vi "Verify File Path.vi"(7 "Default Path":path, 8 "error in":errorcluster, 11 "File Name or Path":string) -> (0 "error out":errorcluster, 3 "File":path, 5 "Stripped Path":path)   [LabVIEW 2021, in "File_CIF_U.lvlib"]
uses:
  File_CIF_U.lvlib
  typedef/File Errors.ctl
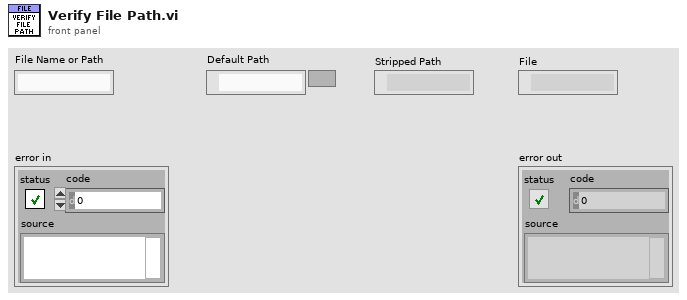
[diagram p1: front panel]
types:
  T1 = typedef "File_CIF_U.lvlib/File Errors.ctl" = enum16{"Invalid File Path"}
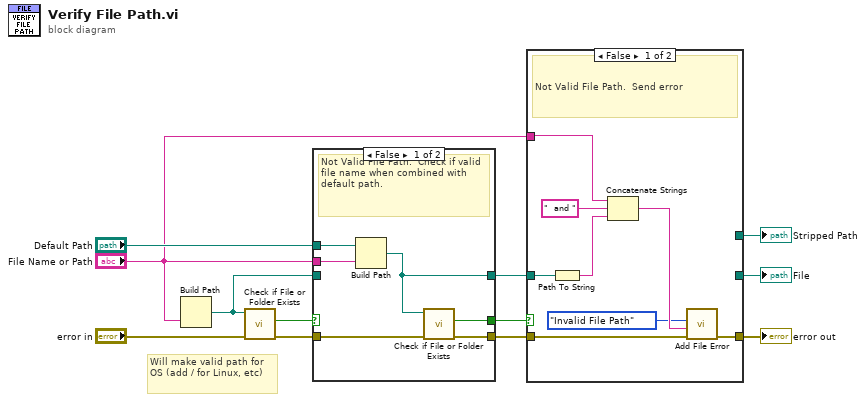
[diagram p0: block diagram]
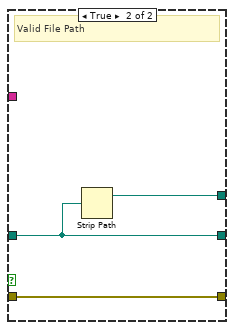
[diagram p2: hidden frame]
diagram:
  # "Will make valid path for OS (add / for Linux, etc)"
  n1 = Build Path(name or relative path="File Name or Path") -> (appended path=w9:path)  [unwired: 1 in]
  n2 = call <vilib>:"Check if File or Folder Exists.vi"("error in (no error)"="error in", "path"=w9) -> ("error out"=w8:errorcluster, "file or folder exists?"=w10:bool)  [unwired: 7 in, 1 out]
  n3 = case shown="False" w10 {
    selector: w10 -> [_ w19]
    tunnel: w9 -> [_ w21]
    tunnel: "File Name or Path" -> [w18 _]
    tunnel: "Default Path" -> [w17 _]
    tunnel: w8 -> [w16 w20]
    tunnel: [w15 w20] -> w7
    tunnel: [w14 w19] -> w6
    tunnel: [w13 w21] -> w5
    frame False {
      # "Not Valid File Path.  Check if valid file name when combined with default path."
      n4 = Build Path(base path=w17, name or relative path=w18) -> (appended path=w13:path)
      n5 = call <vilib>:"Check if File or Folder Exists.vi"("error in (no error)"=w16, "path"=w13) -> ("error out"=w15:errorcluster, "file or folder exists?"=w14:bool)  [unwired: 7 in, 1 out]
    }
    frame True {
      # "Valid File Path"
    }
  }
  n6 = case shown="False" w6 {
    tunnel: w5 -> [w27 w31]
    tunnel: w7 -> [w29 w32]
    tunnel: [w28 w32] -> w1
    tunnel: [_ w31] -> w4
    tunnel: [_ w30] -> w3
    tunnel: "File Name or Path" -> [w26 _]
    frame False {
      # "Not Valid File Path.  Send error"
      n7 = Path To String(path=w27) -> (string=w24:string)
      n8 = Concatenate Strings(w26, "  and " ("string"), w24) -> (w23:string)
      n9 = call "Add File Error.vi"("error in (no error)"=w29, "String to Append"=w23, "Error"=File_Errors."Invalid File Path") -> ("error out"=w28:errorcluster)  [unwired: 8 in]
    }
    frame True {
      # "Valid File Path"
      n10 = Strip Path(path=w31) -> (stripped path=w30:path)  [unwired: 1 out]
    }
  }
  "File" <- w4
  "Stripped Path" <- w3
  "error out" <- w1
